vi "Get qd Temp (rotate and normal) (SubVI).vi"(10 "Instrument Type":T1=enum."SVSM", 11 ".NET引用句柄输入":refnum<k24>) -> (3 "Temperature":dbl)   [LabVIEW 2019, in "SubVI.lvlib"]
uses:
  SubVI.lvlib
  lib/QDInstrument.dll
  Instrument Type.ctl
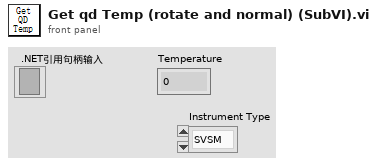
[diagram p1: front panel]
types:
  T1 = typedef "Instrument Type.ctl" = enum16{"PPMS", "VersaLab", "DynaCool", "SVSM", "PPMS-Rotate", "Lakeshore335", "9T mag"}
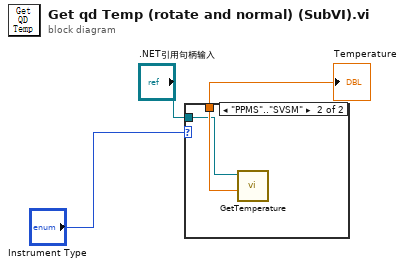
[diagram p0: block diagram]
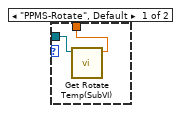
[diagram p2: hidden frame]
diagram:
  n1 = case shown="\"PPMS\"..\"SVSM\"" "Instrument Type" {
    tunnel: [w4 w7] -> w2
    tunnel: ".NET引用句柄输入" -> [w5 w6]
    frame "PPMS-Rotate", Default {
      n2 = call "Get Rotate Temp(SubVI).vi"(".NET引用句柄输入"=w5) -> ("Result"=w4:dbl)  [unwired: 10 in]
    }
    frame "PPMS".."SVSM" {
      n3 = call "GetTemperature.vi"("Instrument Ref In"=w6) -> ("Temperature"=w7:dbl)  [unwired: 4 in, 4 out]
    }
  }
  "Temperature" <- w2
